vi "Get Settings.vi"(8 "error in (no error)":errorcluster, 11 "Cryo-Con Driver in":refnum<class "Cryo-Con Driver.lvclass">) -> (0 "error out":errorcluster, 2 "Settings":string[](array[string]), 3 "Cryo-Con Driver out":refnum<class "Cryo-Con Driver.lvclass">)   [LabVIEW 2021, in "Cryo-Con Driver.lvclass"]
uses:
  Cryo-Con Driver.lvclass
  C:/GitHub/NHMFL_Core/Libraries/Instruments/VISA Instrument/VISA Instrument.lvclass
  C:/GitHub/NHMFL_Core/Libraries/Instruments/Temperature Controller Driver/Temperature Controller Driver.lvclass
  C:/GitHub/NHMFL_Core/Libraries/Instruments/Instrument Driver/Instrument Driver.lvclass
  VISA Instrument/VISA Instrument.lvclass/VISA Instrument.ctl
  Instrument Driver/Instrument Driver.lvclass/Instrument Driver.ctl
  VISA Instrument/Write VISA resource.vi
  VISA Instrument/Read VISA resource.vi
  Instrument Driver/Read Recorder name.vi
  Temperature Controller Driver/Read T controller configuration.vi
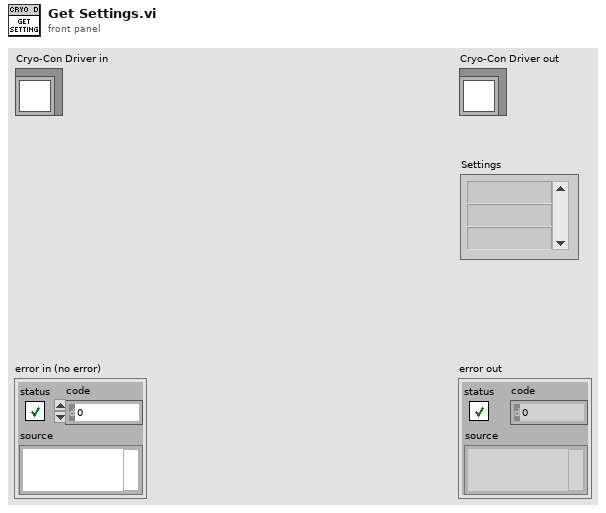
[diagram p1: front panel]
types:
  T1 = typedef "T controller configuration.ctl" = cluster{"Record Channels":string[], "Record raw signal":bool, "Set point":dbl, "Record heater":bool, "Ramp rate":dbl, "P":dbl, "I":dbl, "D":dbl, "Control":T2, "P manual":dbl, "Output #":i32}
  T2 = typedef "Control Mode.ctl" = enum16{"Off", "PID", "Ramp", "Manual", "Table"}
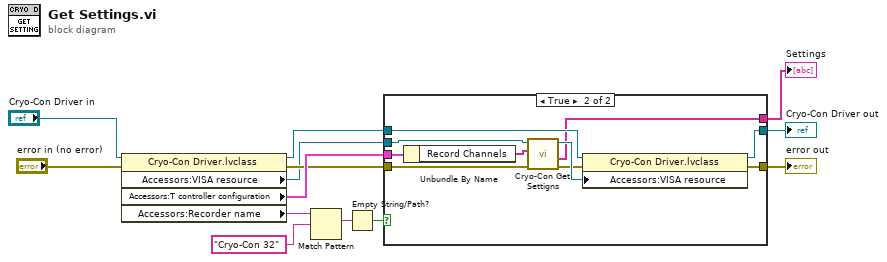
[diagram p0: block diagram]
diagram:
  n1 = property class="Cryo-Con Driver.lvclass"(reference="Cryo-Con Driver in", error in="error in (no error)") -> (reference out=w6:refnum<class "Cryo-Con Driver.lvclass">, error out=w8:errorcluster, "Accessors:VISA resource"=w7:refnum<visa-resource-name>, "Accessors:T controller configuration"=w9:T1, "Accessors:Recorder name"=w10:string)
  n2 = Match Pattern(string=w10, regular expression="Cryo-Con 32") -> (match substring=w12:string)  [unwired: 1 in, 3 out]
  n3 = Empty String/Path?(string/path=w12) -> (empty?=w13:bool)
  n4 = case shown="True" w13 {
    tunnel: [w14 w25] -> w2
    tunnel: w6 -> [w15 w24]
    tunnel: [w15 w23] -> w3
    tunnel: w7 -> [_ w22]
    tunnel: w8 -> [w14 w20]
    tunnel: w9 -> [_ w18]
    tunnel: [_ w16] -> w1
    frame False {
    }
    frame True {
      n5 = Unbundle By Name(w18) -> ("Record Channels"=w17:string[])
      n6 = call "Cryo-Con Get Settigns.vi"("Error In"=w20, "Inputs"=w17, "VISA resource name"=w22) -> ("Error Out"=w19:errorcluster, "Settings"=w16:string[], "VISA resource name out"=w21:refnum<visa-resource-name>)  [unwired: 6 in]
      n7 = property class="Cryo-Con Driver.lvclass"(reference=w24, error in=w19, "Accessors:VISA resource"=w21) -> (reference out=w23:refnum<class "Cryo-Con Driver.lvclass">, error out=w25:errorcluster)
    }
  }
  "error out" <- w2
  "Cryo-Con Driver out" <- w3
  "Settings" <- w1
